vi "Teleop.vi"(10 "Match Info":T2={"Autonomous Elapsed Seconds"=0.0, "TeleOp Elapsed Seconds"=0.0, "Disabled Elapsed Seconds"=0.0, "Visited Autonomous"=FALSE, "Visited TeleOp"=FALSE, "Visited Disabled"=FALSE, "Autonomous Settings"={"Autonomous Style"=enum."Independent", "VI Refnum"=refnum}}, 11 "Call Context":T3) -> ()   [LabVIEW 2017]
doc: "This VI is called for each TeleOp packet received from the DS where the robot is not disabled. It is often used to read from the joysticks and update I/O or to update setpoints for timed control loops. It should complete and return within 20 milliseconds or it may miss DS packets."
uses:
  <vilib>/Rock Robotics/WPI/DriverStation/WPI_DriverStationDerivedRobotMode.ctl
  <vilib>/Rock Robotics/WPI/DriverStation/WPI_DriverStationMatch Info.ctl
  <vilib>/Rock Robotics/WPI/Solenoid/WPI_SolenoidValue.ctl
  <vilib>/Rock Robotics/WPI/Utilities/WPI_GetSetVariantRefNum.vi
  <vilib>/Rock Robotics/Network Tables/NT Write Boolean Array.vi
  <vilib>/Rock Robotics/Network Tables/NT Write Numeric Array.vi
  <vilib>/Rock Robotics/Network Tables/NT Read Boolean.vi
  <vilib>/Rock Robotics/Network Tables/NT Read Number.vi
  <vilib>/Rock Robotics/WPI/Solenoid/WPI_SolenoidSetEnum.vi
panel:
  out "Buttons":bool[](array[boolean])
  out "Axes":dbl[](array[numeric])
  out "Compressor Error":errorcluster
  out "Compressor Enabled?":bool
  out "Compressor Running?":bool
  out "Current Solenoid Output":T1
  out "Solenoid Errors":errorcluster
  out "Climb Motor Errors":errorcluster
  out "Climb Motor Output":dbl
  out "Sample Slider 0":dbl(slide) scale=0.0..5.0
  out "Sample Boolean 1":bool
  out "Sample Boolean 0":bool
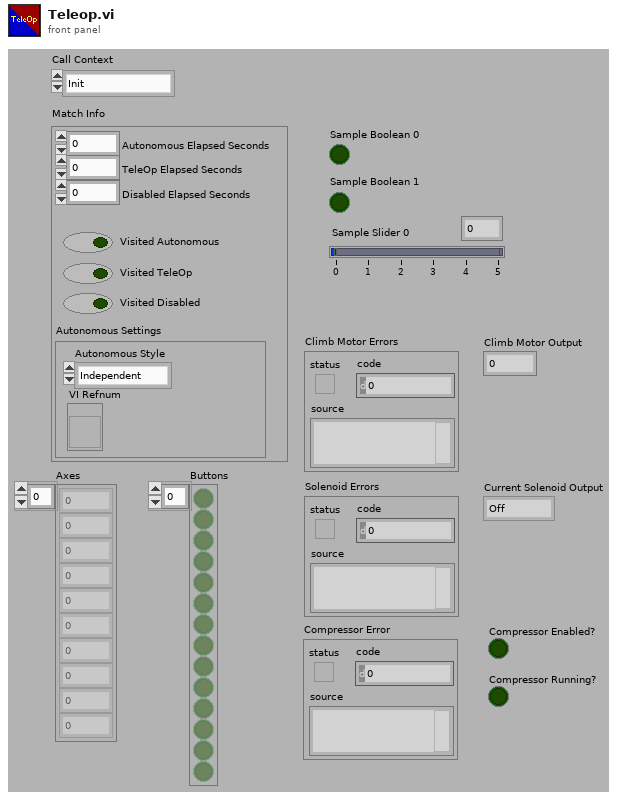
[diagram p1: front panel]
types:
  T1 = typedef "WPI_SolenoidValue.ctl" = enum16{"Off", "On", "Forward", "Reverse"}
  T2 = typedef "WPI_DriverStationMatch Info.ctl" = cluster{"Autonomous Elapsed Seconds":dbl, "TeleOp Elapsed Seconds":dbl, "Disabled Elapsed Seconds":dbl, "Visited Autonomous":bool, "Visited TeleOp":bool, "Visited Disabled":bool, "Autonomous Settings":cluster{"Autonomous Style":enum16{"Iterative", "Independent"}, "VI Refnum":refnum<vi>}}
  T3 = typedef "WPI_DriverStationDerivedRobotMode.ctl" = enum16{"Init", "Execute", "Stop"}
  T4 = typedef "WPI_JoystickDevRef.ctl" = cluster{"Device":T5}
  T5 = typedef "WPI_JoystickDeviceEnum.ctl" = enum16{"USB 0", "USB 1", "USB 2", "USB 3", "USB 4", "USB 5"}
  T6 = typedef "WPI_RobotDriveDevRef.ctl" = cluster{"DevStatus":errorcluster, "Motors[]":T7[], "Square Inputs":bool, "Max Output":dbl}
  T7 = typedef "WPI_MotorControlDeviceRef.ctl" = cluster{"DeviceStatus":errorcluster, "Type":T8, "PWM":cluster{"PWM Channel":T9, "DeadBand":T10}, "CAN":cluster{"Device Number":u8, "SetOutput VI Ref":variant, "GetOutput VI Ref":variant, "Enable VI Ref":variant, "Disable VI Ref":variant, "Data":variant}, "Invert":bool, "DIO PWM":cluster{"PWM \"Enable\" Channel":T9, "DIOChannel":T11, "PWM Rate":dbl}}
  T8 = typedef "WPI_MotorControlType.ctl" = enum16{"PWM", "CAN", "DIO PWM"}
  T9 = typedef "FPGA_DIOPWMChannel.ctl" = enum8{"PWM 0", "PWM 1", "PWM 2", "PWM 3", "PWM 4", "PWM 5", "PWM 6", "PWM 7", "PWM 8", "PWM 9", "PWM MXP 0", "PWM MXP 1", "PWM MXP 2", "PWM MXP 3", "PWM MXP 4", "PWM MXP 5", "PWM MXP 6", "PWM MXP 7", "PWM MXP 8", "PWM MXP 9", "Invalid"}
  T10 = typedef "WPI_PWMDeadband.ctl" = cluster{"Name":string, "maxPositivePwm":i32, "minPositivePwm":i32, "centerPwm":i32, "maxNegativePwm":i32, "minNegativePwm":i32, "angularRange":u16}
  T11 = typedef "FPGA_DIOChannel.ctl" = enum8{"DIO 0", "DIO 1", "DIO 2", "DIO 3", "DIO 4", "DIO 5", "DIO 6", "DIO 7", "DIO 8", "DIO 9", "DIO MXP 0", "DIO MXP 1", "DIO MXP 2", "DIO MXP 3", "DIO MXP 4", "DIO MXP 5", "DIO MXP 6", "DIO MXP 7", "DIO MXP 8", "DIO MXP 9", "DIO MXP 10", "DIO MXP 11", "DIO MXP 12", "DIO MXP 13", "DIO MXP 14", "DIO MXP 15", "SPI Port CS1", "SPI Port CS2", "SPI Port CS3", "SPI Port MISO", "SPI Port MOSI", "Invalid"}
  T12 = typedef "WPI_CompressorDevRef.ctl" = cluster{"DevStatus":errorcluster, "Pneumatics Control Module":u8}
  T13 = typedef "WPI_SolenoidDevRef.ctl" = cluster{"DevStatus":errorcluster, "Pneumatics Control Module":u8, "Forward Solenoid Channel":T14, "Reverse Solenoid Channel":T14}
  T14 = typedef "WPI_SolenoidChannel.ctl" = enum8{"Solenoid 0", "Solenoid 1", "Solenoid 2", "Solenoid 3", "Solenoid 4", "Solenoid 5", "Solenoid 6", "Solenoid 7", "Invalid"}
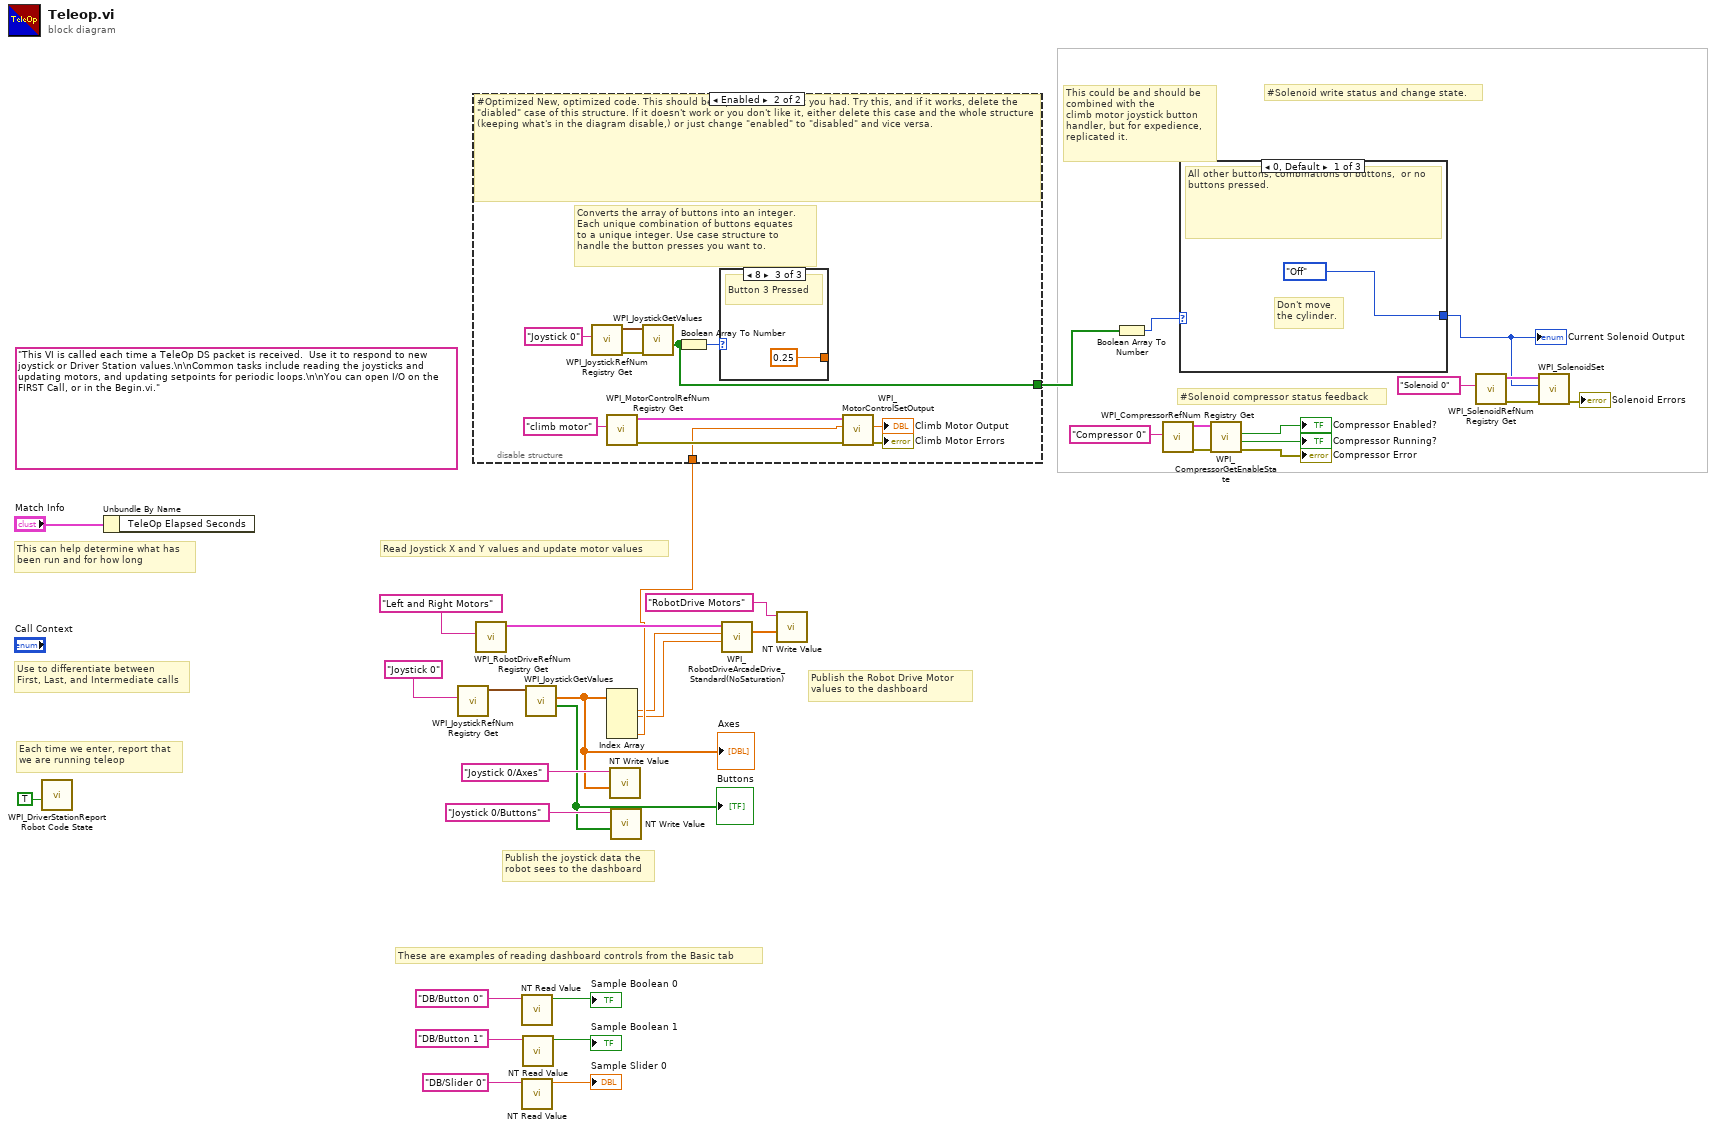
[diagram p0: block diagram]
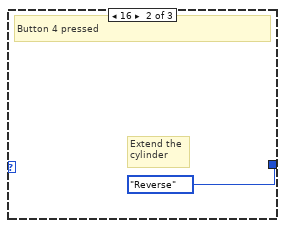
[diagram p2: hidden frame]
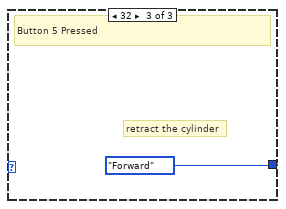
[diagram p3: hidden frame]
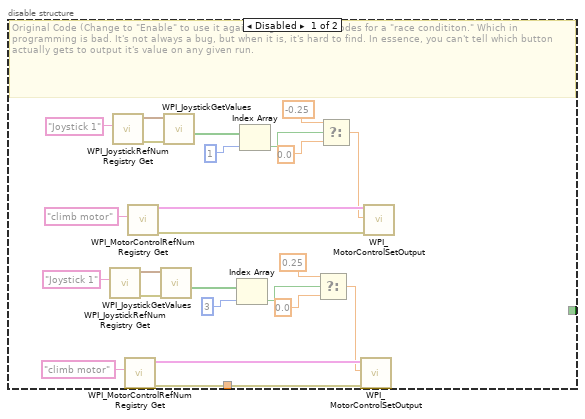
[diagram p4: hidden frame]
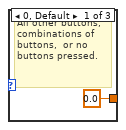
[diagram p5: hidden frame]
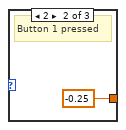
[diagram p6: hidden frame]
diagram:
  (unwired) "This VI is called each time a TeleOp DS packet is received.  Use it to respond to new joystick or Driver Station values.\n\nCommon tasks include reading the joysticks and updating motors, and updating setpoints for periodic loops.\n\nYou can open I/O on the FIRST Call, or in the Begin.vi."
  # "#Solenoid compressor status feedback"
  # "#Solenoid write status and change state."
  # "This could be and should be\ncombined with the \nclimb motor joystick button\nhandler, but for expedience,\nreplicated it."
  # "These are examples of reading dashboard controls from the Basic tab"
  # "Publish the Robot Drive Motor\nvalues to the dashboard"
  # "Publish the joystick data the\nrobot sees to the dashboard"
  # "Each time we enter, report that\nwe are running teleop"
  # "Use to differentiate between\nFirst, Last, and Intermediate calls"
  # "This can help determine what has\nbeen run and for how long"
  # "Read Joystick X and Y values and update motor values"
  n1 = call <vilib>:"WPI_DriverStationReport Robot Code State.vi"("TeleOp"=TRUE ("Autonomous")) -> ()  [unwired: 10 in, 1 out]
  n2 = Unbundle By Name("Match Info") -> ()  [unwired: 1 out]
  n3 = call <vilib>:"WPI_JoystickRefNum Registry Get.vi"("refnum name"="Joystick 0") -> ("JoystickDevRef"=w4:T4)  [unwired: 1 in, 9 out]
  n4 = call <vilib>:"WPI_RobotDriveRefNum Registry Get.vi"("refnum name"="Left and Right Motors") -> ("RobotDriveDevRef"=w32:T6)  [unwired: 1 in, 9 out]
  n5 = call-poly <vilib>:"NT Read Value.vi"("Name"="DB/Button 0" ("refnum name")) -> ("Boolean"=→"Sample Boolean 0":bool)  [unwired: 9 in, 1 out]
  n6 = call-poly <vilib>:"NT Read Value.vi"("Name"="DB/Slider 0" ("refnum name")) -> ("Numeric"=→"Sample Slider 0":dbl)  [unwired: 9 in, 1 out]
  n7 = call-poly <vilib>:"NT Read Value.vi"("Name"="DB/Button 1" ("refnum name")) -> ("Boolean"=→"Sample Boolean 1":bool)  [unwired: 9 in, 1 out]
  n8 = call <vilib>:"WPI_JoystickGetValues.vi"("JoystickDevRef"=w4) -> ("Buttons"=w26:bool[], "Axes"=w27:dbl[])  [unwired: 6 in, 3 out]
  "Axes" <- w27
  "Buttons" <- w26
  n9 = Index Array(array=w27) -> (element #1=w1:dbl, element #2=w2:dbl, element #4=w3:dbl)  [unwired: 4 in, 1 out]
  n10 = disable-structure shown="Enabled" {
    disable-tunnel: [_ w62] -> w14
    disable-tunnel: w3 -> [_ w59]
    frame Disabled {
      # "Original Code (Change to \"Enable\" to use it again.) Right now, this codes for a \"race condititon.\" Which in programming is bad. It's not always a bug, but when it is, it's hard to find. In essence, you can't tell which button actually gets to output it's value on any given run."
      n11 = call <vilib>:"WPI_JoystickRefNum Registry Get.vi"("refnum name"="Joystick 1") -> ("error out"=w54:errorcluster, "JoystickDevRef"=w55:T4)  [unwired: 9 in]
      n12 = call <vilib>:"WPI_JoystickRefNum Registry Get.vi"("refnum name"="Joystick 1") -> ("error out"=w42:errorcluster, "JoystickDevRef"=w43:T4)  [unwired: 9 in]
      n13 = call <vilib>:"WPI_MotorControlRefNum Registry Get.vi"("refnum name"="climb motor") -> ("error out"=w57:errorcluster, "MotorControlDevRef"=w58:T7)  [unwired: 9 in]
      n14 = call <vilib>:"WPI_MotorControlRefNum Registry Get.vi"("refnum name"="climb motor") -> ("error out"=w45:errorcluster, "MotorControlDevRef"=w46:T7)  [unwired: 9 in]
      n15 = call <vilib>:"WPI_JoystickGetValues.vi"("error in (no error)"=w54, "JoystickDevRef"=w55) -> ("Buttons"=w52:bool[])  [unwired: 5 in, 4 out]
      n16 = call <vilib>:"WPI_JoystickGetValues.vi"("error in (no error)"=w42, "JoystickDevRef"=w43) -> ("Buttons"=w40:bool[])  [unwired: 5 in, 4 out]
      n17 = Index Array(array=w52, index=3) -> (element=w48:bool)
      n18 = Index Array(array=w40, index=1) -> (element=w36:bool)
      n19 = Select(t=0.25, s=w48, f=0.0) -> (s? t:f=w47:dbl)
      n20 = Select(t=-0.25, s=w36, f=0.0) -> (s? t:f=w35:dbl)
      n21 = call <vilib>:"WPI_MotorControlSetOutput.vi"("error in (no error)"=w57, "Output"=w47, "MotorControlDevRef"=w58) -> ()  [unwired: 6 in, 3 out]
      n22 = call <vilib>:"WPI_MotorControlSetOutput.vi"("error in (no error)"=w45, "Output"=w35, "MotorControlDevRef"=w46) -> ()  [unwired: 6 in, 3 out]
    }
    frame Enabled {
      # "Converts the array of buttons into an integer.\nEach unique combination of buttons equates\nto a unique integer. Use case structure to \nhandle the button presses you want to."
      # "#Optimized New, optimized code. This should be equivalent to what you had. Try this, and if it works, delete the \"diabled\" case of this structure. If it doesn't work or you don't like it, either delete this case and the whole structure (keeping what's in the diagram disable,) or just change \"enabled\" to \"disabled\" and vice versa."
      n23 = call <vilib>:"WPI_JoystickRefNum Registry Get.vi"("refnum name"="Joystick 0") -> ("error out"=w69:errorcluster, "JoystickDevRef"=w68:T4)  [unwired: 9 in]
      n24 = call <vilib>:"WPI_MotorControlRefNum Registry Get.vi"("refnum name"="climb motor") -> ("error out"=w67:errorcluster, "MotorControlDevRef"=w66:T7)  [unwired: 9 in]
      n25 = call <vilib>:"WPI_JoystickGetValues.vi"("error in (no error)"=w69, "JoystickDevRef"=w68) -> ("Buttons"=w62:bool[])  [unwired: 5 in, 4 out]
      n26 = Boolean Array To Number(Boolean array=w62) -> (number=w63:u32)
      n27 = case shown="8" w63 {
        tunnel: [0.0 -0.25 0.25] -> _
        frame 0, Default {
          # "All other buttons, combinations of buttons,  or no buttons pressed."
        }
        frame 2 {
          # "Button 1 pressed"
        }
        frame 8 {
          # "Button 3 Pressed"
        }
      }
      n28 = call <vilib>:"WPI_MotorControlSetOutput.vi"("error in (no error)"=w67, "Output"=w59, "MotorControlDevRef"=w66) -> ("error out"=→"Climb Motor Errors":errorcluster, "Motor Output"=→"Climb Motor Output":dbl)  [unwired: 6 in, 1 out]
    }
  }
  n29 = call-poly <vilib>:"NT Write Value.vi"("Numeric Array"=w27, "Name"="Joystick 0/Axes") -> ()  [unwired: 9 in, 1 out]
  n30 = call-poly <vilib>:"NT Write Value.vi"("Boolean Array"=w26, "Name"="Joystick 0/Buttons") -> ()  [unwired: 9 in, 1 out]
  n31 = call <vilib>:"WPI_RobotDriveArcadeDrive_Standard(NoSaturation).vi"("Y axis value"=w2, "X axis value"=w1, "RobotDriveDevRef"=w32) -> ("Motor Values"=w19:dbl[])  [unwired: 1 in, 7 out]
  n32 = call-poly <vilib>:"NT Write Value.vi"("Numeric Array"=w19, "Name"="RobotDrive Motors") -> ()  [unwired: 9 in, 1 out]
  n33 = Boolean Array To Number(Boolean array=w14) -> (number=w6:u32)
  n34 = call <vilib>:"WPI_CompressorRefNum Registry Get.vi"("refnum name"="Compressor 0") -> ("error out"=w11:errorcluster, "CompressorDevRef"=w10:T12)  [unwired: 9 in]
  n35 = case shown="0, Default" w6 {
    tunnel: [WPI_SolenoidValue."Off" ("Value") WPI_SolenoidValue."Reverse" ("Value") WPI_SolenoidValue."Forward" ("Value")] -> w5
    frame 0, Default {
      # "Don't move\nthe cylinder."
      # "All other buttons, combinations of buttons,  or no buttons pressed."
    }
    frame 16 {
      # "Extend the \ncylinder"
      # "Button 4 pressed"
    }
    frame 32 {
      # "retract the cylinder"
      # "Button 5 Pressed"
    }
  }
  "Current Solenoid Output" <- w5
  n36 = call <vilib>:"WPI_CompressorGetEnableState.vi"("error in (no error)"=w11, "CompressorDevRef"=w10) -> ("error out"=→"Compressor Error":errorcluster, "Compressor Running"=→"Compressor Running?":bool, "Enabled"=→"Compressor Enabled?":bool)  [unwired: 6 in, 1 out]
  n37 = call <vilib>:"WPI_SolenoidRefNum Registry Get.vi"("refnum name"="Solenoid 0") -> ("error out"=w17:errorcluster, "SolenoidDevRef"=w16:T13)  [unwired: 9 in]
  n38 = call-poly <vilib>:"WPI_SolenoidSet.vi"("error in (no error)"=w17, "Value"=w5, "SolenoidDevRef"=w16) -> ("error out"=→"Solenoid Errors":errorcluster)  [unwired: 8 out]
